vi "Orifice coefficient For Air.vi"(0 "RH":dbl min=0.0 max=100.0, 1 "Gas Temperature":dbl[unit]=10.0 min=10.0 max=95.0, 3 "Orifice Diameter":dbl[unit], 4 "Pipe Diameter (mm)":dbl[unit], 5 "P1\n(Presure After Fan &\n before Orifice)":dbl[unit]=80000.0 min=80000.0 max=120000.0, 6 "Delta P\n(Presure Made By Orifice)":dbl[unit]) -> (7 "Iteration Volumetric Flow \n(Orifice) (m^3/s)":dbl[unit], 8 "Mass Flow (Orifice) (Kg/s)":dbl[unit])   [LabVIEW 2018]
panel:
  out "Mass Flow (Orifice) (Kg/h)":dbl[unit]
  out "Mass Flow (Orifice) (Kg/h)":dbl[unit](knob)
  out "ReD":dbl
  out "Gas Viscosity\nof Humid Air":dbl[unit]
  out "Pipe Velocity (m/s)":dbl[unit]
  out "Pipe Area (m^2)":dbl[unit]
  out "Throat Velocity (m/s)":dbl[unit]
  out "Throat Area (m^2)":dbl[unit]
  out "Beta":dbl
  out "Pipe Diameter (inch)":dbl[unit]
  out "orifice coefficient":dbl
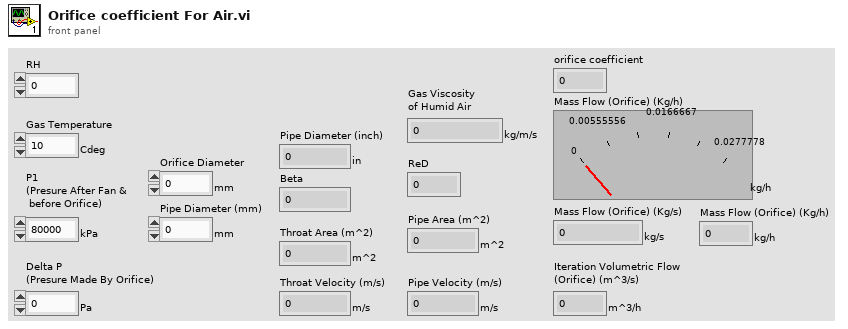
[diagram p1: front panel]
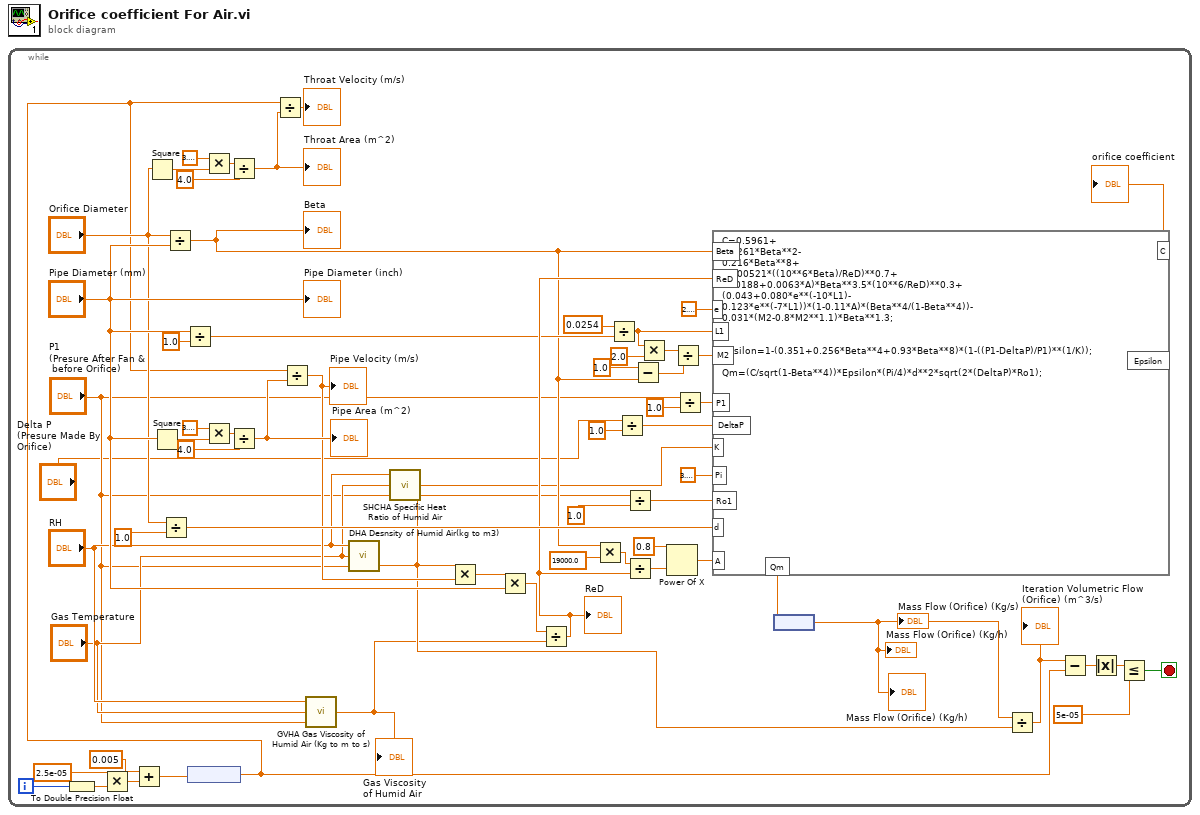
[diagram p0: block diagram]
diagram:
  n1 = while {
    i -> [w18]
    stop <- w12 stop-if-true
    n2 = To Double Precision Float(number=w18) -> (double precision float=w22:dbl)
    n3 = Multiply(x=2.5e-05, y=w22) -> (x*y=w20:dbl)
    n4 = Add(x=0.005, y=w20) -> (x+y=w17:dbl)
    n5 = Square(x="Orifice Diameter") -> (x^2=w58:dbl[unit])
    n6 = Square(x="Pipe Diameter (mm)") -> (x^2=w54:dbl[unit])
    n7 = Divide(x="Orifice Diameter", y=dbl[unit] 1.0) -> (x/y=w50:dbl)
    n8 = Divide(x="Orifice Diameter", y="Pipe Diameter (mm)") -> (x/y=w26:dbl)
    "Beta" <- w26
    n9 = Divide(x="Pipe Diameter (mm)", y=dbl[unit] 1.0) -> (x/y=w37:dbl)
    n10 = node(w17) -> (w16:dbl[unit])
    n11 = Multiply(x=3.141592653589793, y=w58) -> (x*y=w60:dbl[unit])
    n12 = Multiply(x=3.141592653589793, y=w54) -> (x*y=w56:dbl[unit])
    n13 = Divide(x=w60, y=4.0) -> (x/y=w62:dbl[unit])
    "Throat Area (m^2)" <- w62
    n14 = Divide(x=w56, y=4.0) -> (x/y=w53:dbl[unit])
    "Pipe Area (m^2)" <- w53
    n15 = Divide(x=w16, y=w62) -> (x/y=→"Throat Velocity (m/s)":dbl[unit])
    n16 = Divide(x=w16, y=w53) -> (x/y=w46:dbl[unit])
    "Pipe Velocity (m/s)" <- w46
    n17 = call "GVHA Gas Viscosity of Humid Air (Kg to m to s).vi"("Gas Presure"="P1\n(Presure After Fan &\n before Orifice)", "Tceg"="Gas Temperature", "RH"="RH") -> ("Gas Viscosity Of  Humid Air"=w6:dbl[unit])
    "Gas Viscosity\nof Humid Air" <- w6
    n18 = call "DHA Desnsity of Humid Air(kg to m3).vi"("Total Pressure of Humid Air"="P1\n(Presure After Fan &\n before Orifice)", "Tceg"="Gas Temperature", "RH"="RH") -> ("DHA"=w11:dbl[unit])
    n19 = call "SHCHA Specific Heat Ratio of Humid Air.vi"("Gas Presure"="P1\n(Presure After Fan &\n before Orifice)", "Tceg"="Gas Temperature", "RH"="RH") -> ("SHRHA"=w25:dbl)
    n20 = Multiply(x=w11, y=w46) -> (x*y=w47:dbl[unit])
    n21 = Multiply(x=w47, y="Pipe Diameter (mm)") -> (x*y=w48:dbl[unit])
    n22 = Divide(x=w48, y=w6) -> (x/y=w43:dbl)
    "ReD" <- w43
    n23 = Multiply(x=w26, y=19000.0) -> (x*y=w44:dbl)
    n24 = Divide(x=0.0254, y=w37) -> (x/y=w36:dbl)
    n25 = Divide(x="Delta P\n(Presure Made By Orifice)", y=dbl[unit] 1.0) -> (x/y=w1:dbl)
    n26 = Divide(x=w11, y=dbl[unit] 1.0) -> (x/y=w31:dbl)
    n27 = Divide(x=w44, y=w43) -> (x/y=w42:dbl)
    n28 = Subtract(x=1.0, y=w26) -> (x-y=w27:dbl)
    n29 = Multiply(x=w36, y=2.0) -> (x*y=w34:dbl)
    n30 = Power Of X(1:w42, 2:0.8 ("y")) -> (0:w40:dbl)
    n31 = Divide(x=w34, y=w27) -> (x/y=w32:dbl)
    n32 = Divide(x="P1\n(Presure After Fan &\n before Orifice)", y=dbl[unit] 1.0) -> (x/y=w10:dbl)
    n33 = formula code="C=0.5961+\n0.0261*Beta**2-\n0.216*Beta**8+\n0.000521*((10**6*Beta)/ReD)**0.7+\n(0.0188+0.0063*A)*Beta**3.5*(10**6/ReD)**0.3+\n(0.043+0.080*e**(-10*L1)-\n0.123*e**(-7*L1))*(1-0.11*A)*(Beta**4/(1-Beta**4))-\n0.031*(M2-0.8*M2**1.1)*Beta**1.3;\n\n\nEpsilon=1-(0.351+0.256*Beta**4+0.93*Beta**8)*(1-((P1-DeltaP)/P1)**(1/K));\n\nQm=(C/sqrt(1-Beta**4))*Epsilon*(Pi/4)*d**2*sqrt(2*(DeltaP)*Ro1);"("Beta"=w26, "ReD"=w43, "A"=w40, "e"=2.718281828459045, "L1"=w36, "M2"=w32, "P1"=w10, "DeltaP"=w1, "K"=w25, "Pi"=3.141592653589793, "Ro1"=w31, "d"=w50) -> ("C"=→"orifice coefficient":dbl, "Qm"=w29:dbl)  [unwired: 1 out]
    n34 = node(w29) -> (w23:dbl[unit])
    "Mass Flow (Orifice) (Kg/s)" <- w23
    "Mass Flow (Orifice) (Kg/h)" <- w23
    "Mass Flow (Orifice) (Kg/h)" <- w23
    n35 = Divide(x=w23, y=w11) -> (x/y=w4:dbl[unit])
    "Iteration Volumetric Flow \n(Orifice) (m^3/s)" <- w4
    n36 = Subtract(x=w4, y=w16) -> (x-y=w15:dbl[unit])
    n37 = Absolute Value(x=w15) -> (abs(x)=w14:dbl[unit])
    n38 = Less Or Equal?(x=w14, y=dbl[unit] 5e-05) -> (x <= y?=w12:bool)
    "Pipe Diameter (inch)" <- "Pipe Diameter (mm)"
  }
